vi "H5Gset_comment.vi"(6 "error in (no error)":errorcluster, 7 "Comment":string, 8 "Name":string, 9 "HDF5 Ref":T1) -> (0 "error out":errorcluster, 3 "HDF5 Ref out":T1)   [LabVIEW 2017]
doc: "Sets comment for specified object."
uses:
  <vilib>/UPVI/lvhdf5/library.llb/HDF5 Ref.ctl
  <vilib>/UPVI/lvhdf5/hdf5.dll
panel:
  # "LVHDF5 Toolkit\nCopyright (c) 2005-2013 by Jason D. Sommerville\nCopyright (c) 2014 by UPVI, LLC.\n\nThis use and distribution of this file is governed by the terms found in \nLICENSE.txt distributed with this toolkit and installed at\n <user.lib>\\_lvhdf5\\LICENSE.txt"
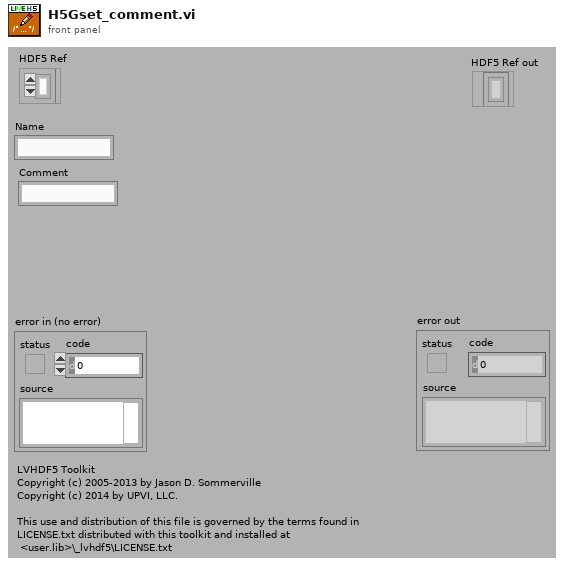
[diagram p1: front panel]
types:
  T1 = typedef "HDF5 Ref.ctl" = refnum<k1>
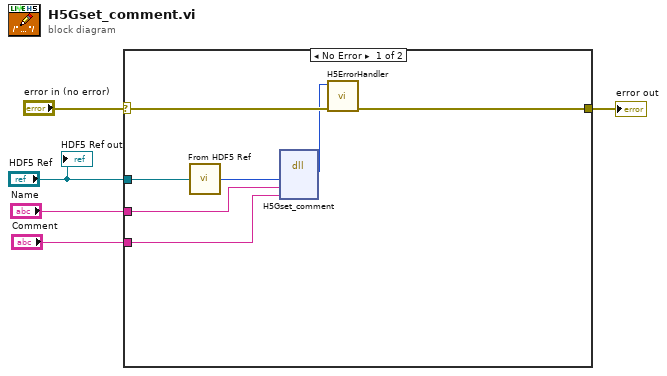
[diagram p0: block diagram]
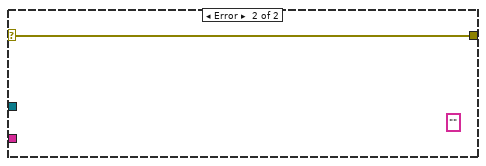
[diagram p2: hidden frame]
diagram:
  n1 = case shown="No Error" "error in (no error)" {
    selector: "error in (no error)" -> [w12 w13]
    tunnel: [w6 w13] -> w4
    tunnel: "HDF5 Ref" -> [w11 _]
    tunnel: "Name" -> [w8 _]
    tunnel: "Comment" -> [w7 _]
    frame No Error {
      n2 = call <vilib>:"From HDF5 Ref.vi"("HDF5 Ref"=w11) -> ("I32"=w10:i32)
      n3 = dll-call lib="C:/Program Files/National Instruments/LabVIEW 2017/vi.lib/UPVI/lvhdf5/hdf5.dll" fn="H5Gset_comment"("loc_id"=w10, "name"=w8, "value"=w7) -> (w9:i32)  [unwired: 6 in, 2 out]
      n4 = call <vilib>:"H5ErrorHandler.vi"("error in (no error)"=w12, "herr_t"=w9) -> ("error out"=w6:errorcluster)  [unwired: 3 in, 4 out]
    }
    frame Error {
      (unwired) "" ("name")
    }
  }
  "error out" <- w4
  "HDF5 Ref out" <- "HDF5 Ref"
